vi "z_disengage_detect_der.vi"(8 "start_der_calc":bool, 10 "z_err":fxp<+/-,24,5>) -> (2 "z_has_disengaged":bool)   [LabVIEW 2017]
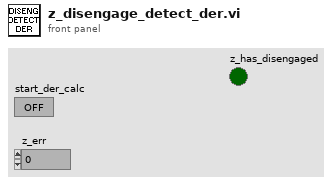
[diagram p1: front panel]
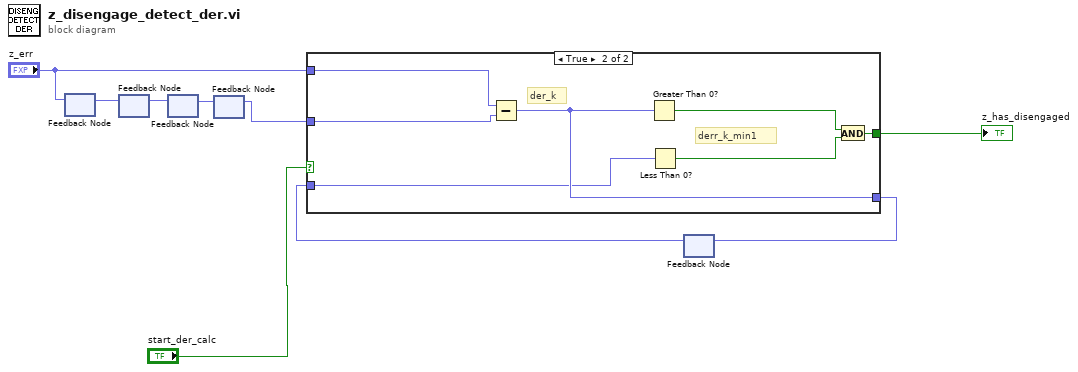
[diagram p0: block diagram]
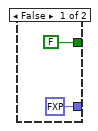
[diagram p2: hidden frame]
diagram:
  n1 = feedback #1() -> (w3:fxp<+/-,24,5>)  [unwired: 1 in]
  n2 = feedback-in #1("z_err") -> ()
  n3 = feedback #2() -> (w4:fxp<+/-,24,5>)  [unwired: 1 in]
  n4 = feedback-in #2(w3) -> ()
  n5 = feedback #3() -> (w5:fxp<+/-,24,5>)  [unwired: 1 in]
  n6 = feedback-in #3(w4) -> ()
  n7 = feedback #4() -> (w1:fxp<+/-,24,5>)  [unwired: 1 in]
  n8 = feedback-in #4(w5) -> ()
  n9 = feedback #5() -> (w6:fxp<+/-,25,6>)  [unwired: 1 in]
  n10 = case shown="True" "start_der_calc" {
    tunnel: "z_err" -> [_ w16]
    tunnel: [FALSE w15] -> w8
    tunnel: [fxp<+/-,25,6> 1.0 w14] -> w7
    tunnel: w6 -> [_ w13]
    tunnel: w1 -> [_ w12]
    frame False {
    }
    frame True {
      # "derr_k_min1"
      # "der_k"
      n11 = Subtract(x=w16, y=w12) -> (x-y=w14:fxp<+/-,25,6>)
      n12 = Greater Than 0?(x=w14) -> (x > 0?=w18:bool)
      n13 = Less Than 0?(x=w13) -> (x < 0?=w17:bool)
      n14 = And(x=w18, y=w17) -> (x .and. y?=w15:bool)
    }
  }
  "z_has_disengaged" <- w8
  n15 = feedback-in #5(w7) -> ()
